vi "Main.vi"() -> ()   [LabVIEW 2018]
uses:
  <vilib>/Instr/_visa.llb/VISA Configure Serial Port (Instr).vi
panel:
  out "Read Count":i32
  out "UART Monitor":string
  out "UART Communication ON/OFF":bool
  in  "VISA resource name":refnum<visa-resource-name>
  in  "Finish Test":bool
  out "Boolean":bool
  in  "Model FLASH Memory":bool
  out "Workspace":string[](array[string])
  out "Tests added to Workspace":i32
  in  "Input":string
  in  "Menu":T1(ring)
  in  "stop":bool
  in  "OK Button":bool
  out "Instructions":string
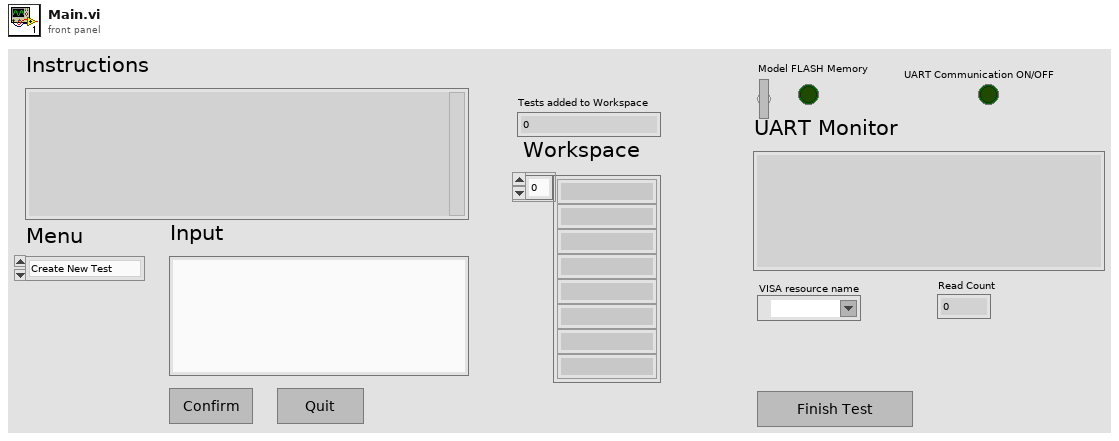
[diagram p1: front panel]
types:
  T1 = enum16{"Create New Test", "Run Single Test", "Run All Tests", "Save Workspace", "Load Workspace", "Delete Test"}
  T2 = enum16{"Inicio", "Create Test A", "Create Test B", "Create Test C", "Create Test D", "Delete Test A", "Delete Test B", "Save", "Load", "Single Test Run", "All Tests Run", "Load Program", "Running Test", "Running Idle", "UART Monitor"}
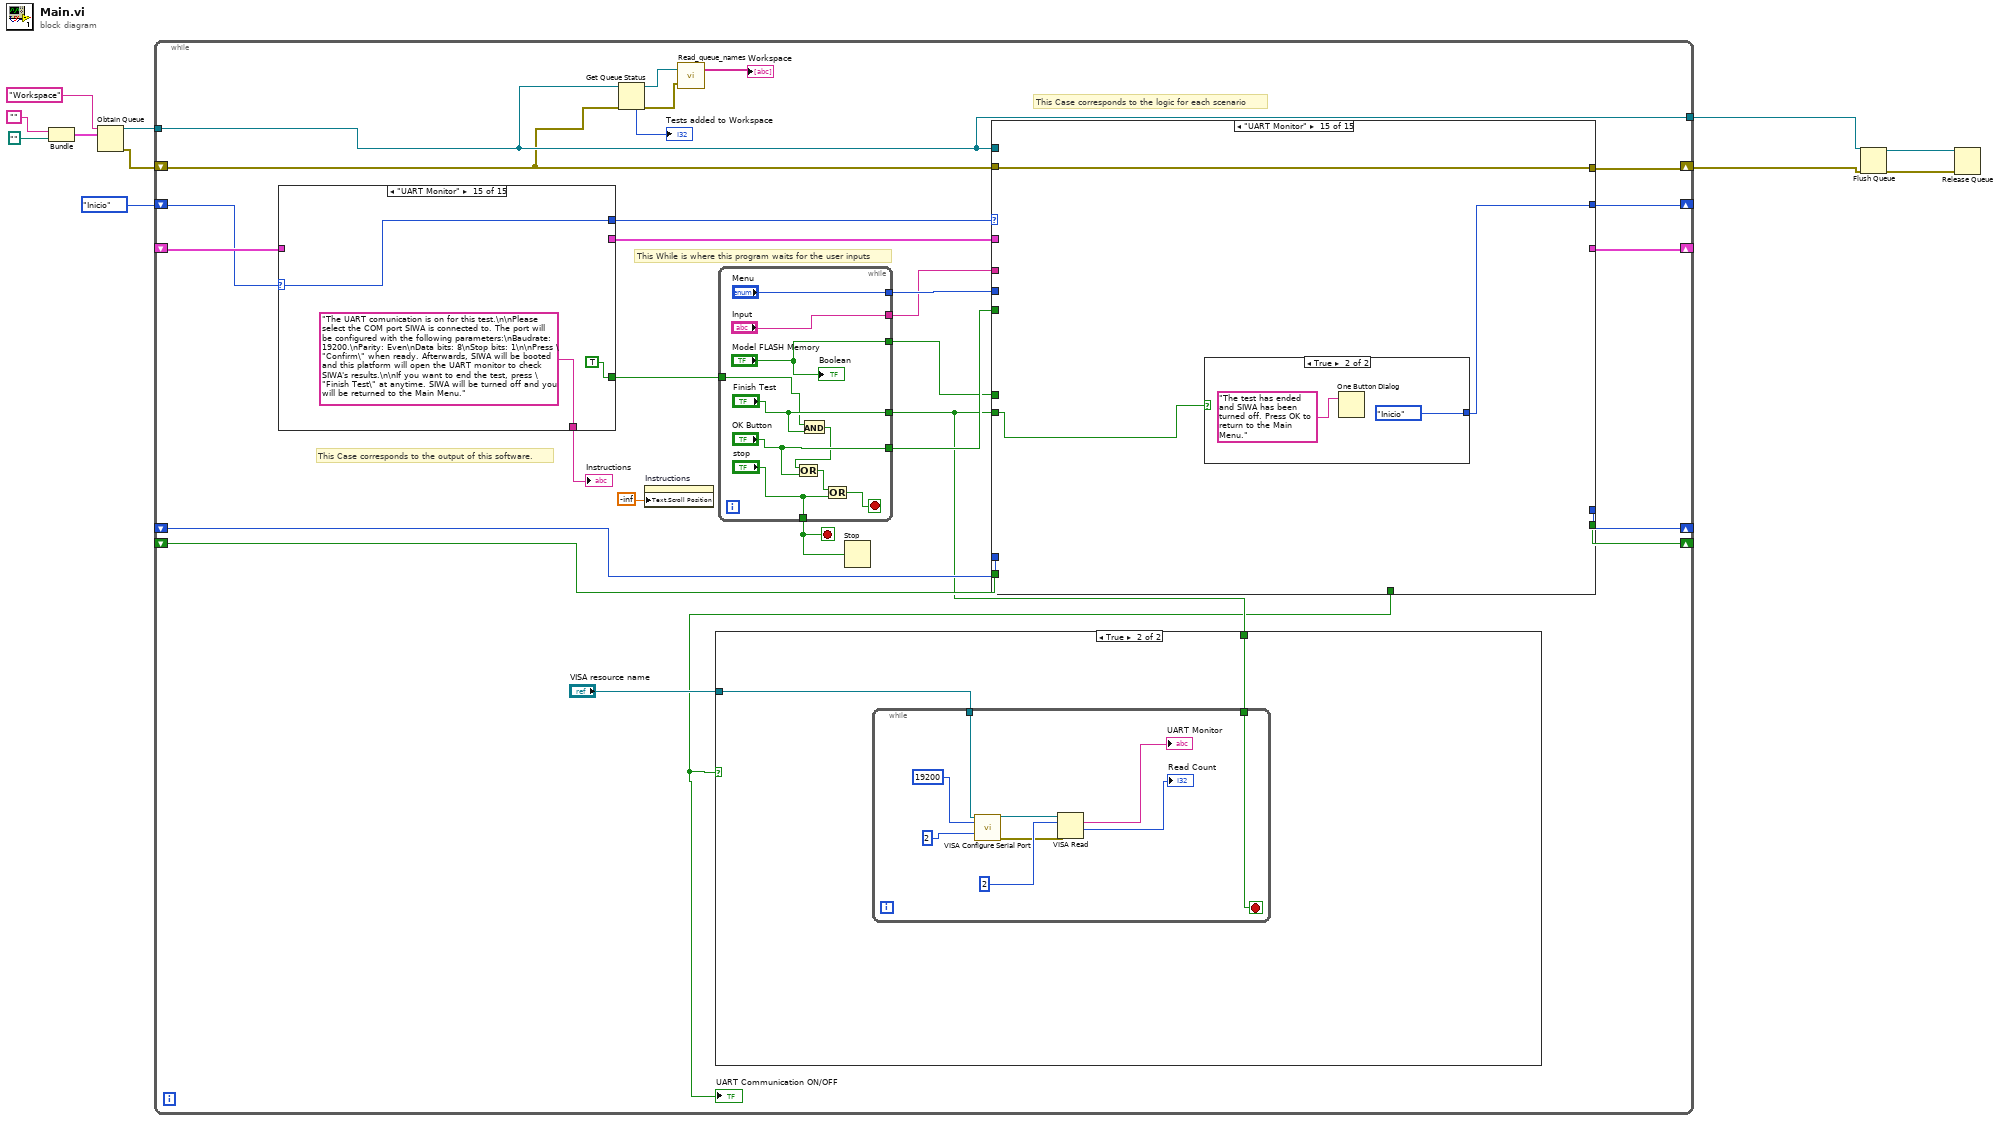
[diagram p0: block diagram]
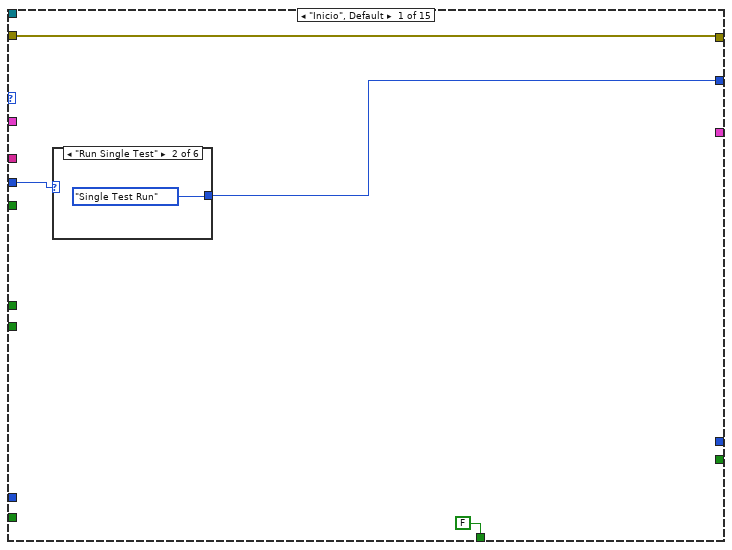
[diagram p3: hidden frame]
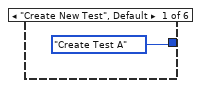
[diagram p4: hidden frame]
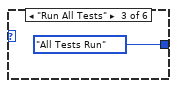
[diagram p5: hidden frame]
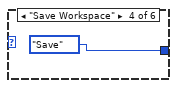
[diagram p6: hidden frame]
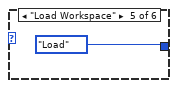
[diagram p7: hidden frame]
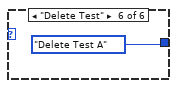
[diagram p8: hidden frame]
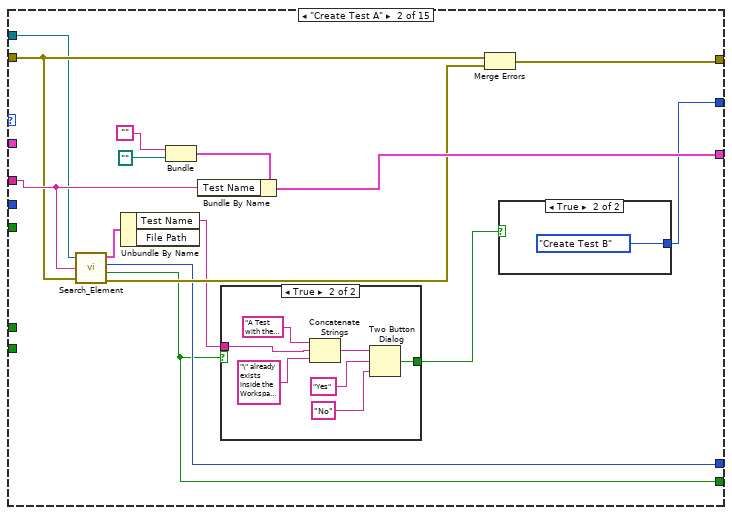
[diagram p9: hidden frame]
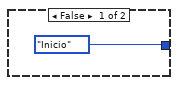
[diagram p10: hidden frame]
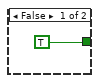
[diagram p11: hidden frame]
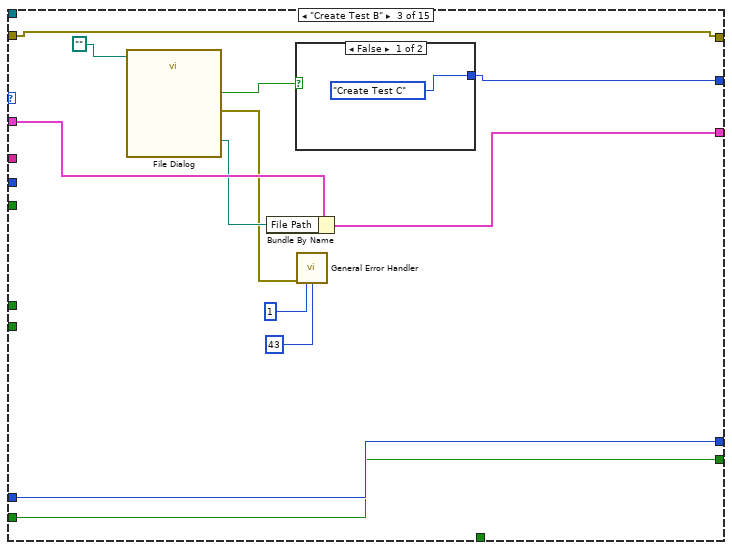
[diagram p12: hidden frame]
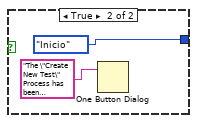
[diagram p13: hidden frame]
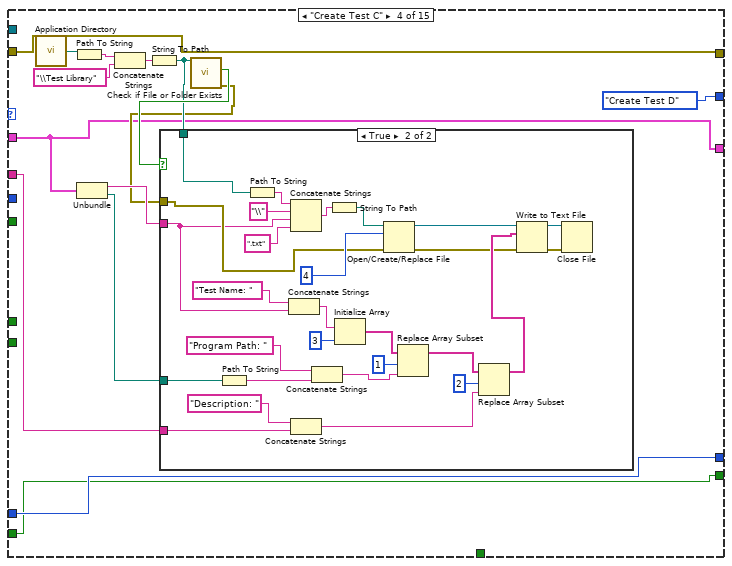
[diagram p14: hidden frame]
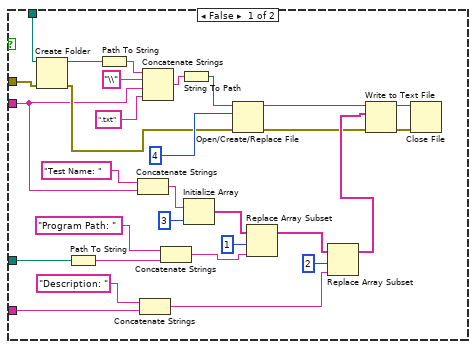
[diagram p15: hidden frame]
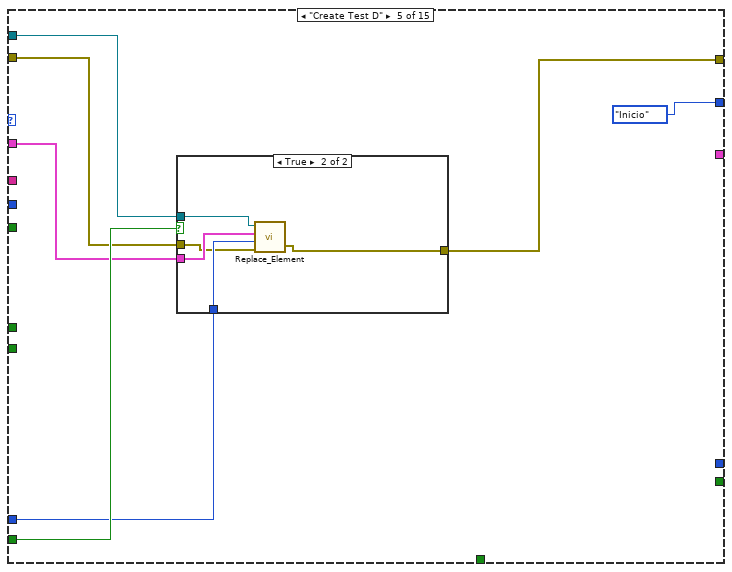
[diagram p16: hidden frame]
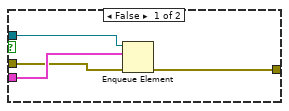
[diagram p17: hidden frame]
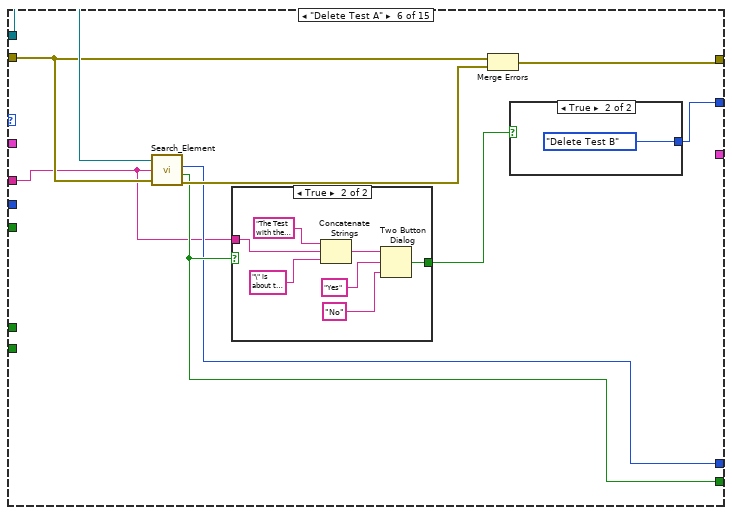
[diagram p18: hidden frame]
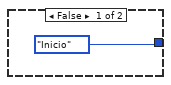
[diagram p19: hidden frame]
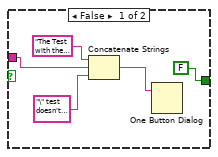
[diagram p20: hidden frame]
diagram:
  n1 = Bundle("Test Name"="", "File Path"=path "") -> (w9:cluster{"Test Name":string, "File Path":path})  [unwired: 1 in]
  n2 = Obtain Queue(name (unnamed)="Workspace", element data type=w9) -> (queue out=w3:refnum<queue>, error out=w7:errorcluster)  [unwired: 3 in, 1 out]
  n3 = while {
    shift-right: [w32] -> _
    shift-left: _ -> [w33]
    shift-right: [w31] -> w6
    shift-left: w7 -> [w25]
    tunnel: w3 -> [w26]
    tunnel: [w26] -> w2
    shift-right: [w24] -> _
    shift-left: _ -> [w23]
    shift-right: [w22] -> _
    shift-left: _ -> [w21]
    shift-right: [w16] -> _
    shift-left: T2."Inicio" -> [w17]
    stop <- w19 stop-if-true
    # "This While is where this program waits for the user inputs"
    # "This Case corresponds to the logic for each scenario"
    # "This Case corresponds to the output of this software."
    n4 = case shown="\"UART Monitor\"" w17 {
      selector: w17 -> [w284 w287 w289 w292 w296 w297 w300 w301 w303 w305 w307 w309 w313 w319 w322]
      tunnel: ["Welcome. This is the Test Environment designed for SIWA.\nSelect which kind of operation do you want to run from the Menu." "Please write below a name for this new test. If the Test File already exists inside the Test Library, it will be overwritted.\n\nThen, press \"Confirm\" to continue." "Now, attach a Program File to this new test. The selected Program File will be the main program loaded in SIWA each time you run this test in the future.\n\nPress \"Confirm\" to continue and select the desired Program File. Press \"OK\" afterwards.\n\nIMPORTANT: The Program File is a .txt file, where each line is a Disassembled 32-bit RISCV Instruction (RV32I format) written in Hexadecimal Code. Please be sure that the selected Program File is constructed in a similar fashion. Otherwise, the test could run into errors." "Write a brief description for this new test.\n\nThe description introduced below will be added to the Test File. That way, it will be easier to understand whatever this test does.\n\nPress Confirm when the description is finished." "The Test File has been created and added to the Testbench succesfully.\n\nYou can find the Test File inside the Test Library folder as <Testname>.txt.\n\nPress Confirm the return to the Main Menu.\n\n" "Introduce the name of the Test you want to remove from the Workspace.\n\nNote: This process won't delete the Test File from your computer. If you wish to delete it completely, it is recommended to do it manually. All tests are stored inside the Test Library file.\n\nPress \"Confirm\" to return to continue." "The selected Test has been succesfully removed from the Workspace.\n\nPress \"Confirm\" to return to the Main Menu." "This feature is still under development.\nPress \"Confirm\" to return to the Main Menu." "This feature is still under development.\nPress \"Confirm\" to return to the Main Menu." "Write the name of the Test you wish to run on SIWA.\n\nPress \"Confirm\" to continue." "This feature is still under development.\nPress \"Confirm\" to return to the Main Menu." "The selected programmed has been loaded inside the FPGA and is ready to be booted on SIWA.\n\nPress \"Confirm\" to boot SIWA.\n\nPress \"Finish Test\" to cancel and return to the Main Menu." "The UART comunication is off for this test. From now on, this platform is indefinitly on an idle state while SIWA is running the loaded program.\n\nIf you want to end the test, press \"Finish Test\". SIWA will be turned off and you will be returned to the Main Menu." w316 "The UART comunication is on for this test.\n\nPlease select the COM port SIWA is connected to. The port will be configured with the following parameters:\nBaudrate: 19200.\nParity: Even\nData bits: 8\nStop bits: 1\n\nPress \"Confirm\" when ready. Afterwards, SIWA will be booted and this platform will open the UART monitor to check SIWA's results.\n\nIf you want to end the test, press \"Finish Test\" at anytime. SIWA will be turned off and you will be returned to the Main Menu."] -> w39
      tunnel: [w284 w287 w289 w292 w296 w297 w300 w301 w303 w305 w307 w309 w313 w319 w322] -> w38
      tunnel: [_ _ w288 w291 w294 _ _ _ _ _ _ _ _ w314 _] -> w34
      tunnel: w33 -> [_ _ w288 w291 w294 _ _ _ _ _ _ _ _ w314 _]
      tunnel: [FALSE _ _ _ _ _ _ _ _ _ _ _ TRUE _ TRUE] -> w12
      frame "Inicio", Default {
      }
      frame "Create Test A" {
      }
      frame "Create Test B" {
      }
      frame "Create Test C" {
      }
      frame "Create Test D" {
      }
      frame "Delete Test A" {
      }
      frame "Delete Test B" {
      }
      frame "Save" {
      }
      frame "Load" {
      }
      frame "Single Test Run" {
      }
      frame "All Tests Run" {
      }
      frame "Running Test" {
      }
      frame "Running Idle" {
      }
      frame "Load Program" {
        n5 = Unbundle By Name(w314) -> ("Test Name"=w315:string)  [unwired: 1 out]
        n6 = Concatenate Strings("The Test with the name \"", w315, "\" test has been selected. The Program File attached to it will be loaded into SIWA.\n\nPress \"Confirm\" to continue.") -> (w316:string)
      }
      frame "UART Monitor" {
      }
    }
    "Instructions" <- w39
    n7 = Get Queue Status(queue=w26, error in (no error)=w25) -> (queue out=w28:refnum<queue>, error out=w20:errorcluster, # elements in queue=→"Tests added to Workspace":i32)  [unwired: 1 in, 5 out]
    n8 = property on="Instructions" class="Str"("Text.Scroll Position"=-inf) -> ()  [unwired: 2 in, 2 out]
    n9 = call "Read_queue_names.vi"("error in (no error)"=w20, "Queue in"=w28) -> ("Array"=→"Workspace":string[])  [unwired: 1 out]
    n10 = while {
      tunnel: ["OK Button"] -> w37
      tunnel: ["stop"] -> w19
      tunnel: ["Menu"] -> w36
      tunnel: ["Input"] -> w35
      tunnel: ["Model FLASH Memory"] -> w18
      tunnel: ["Finish Test"] -> w14
      tunnel: w12 -> [w274]
      stop <- w282 stop-if-true
      n11 = And(x=w274, y="Finish Test") -> (x .and. y?=w273:bool)
      n12 = Or(x=w273, y="OK Button") -> (x .or. y?=w276:bool)
      n13 = Or(x=w276, y="stop") -> (x .or. y?=w282:bool)
      "Boolean" <- "Model FLASH Memory"
    }
    n14 = Stop(stop? (T)=w19) -> ()
    n15 = case shown="\"UART Monitor\"" w38 {
      tunnel: w37 -> [_ _ _ _ _ _ _ _ _ _ _ _ _ _ _]
      tunnel: w36 -> [w54 _ _ _ _ _ _ _ _ _ _ _ _ _ _]
      tunnel: w35 -> [_ w71 _ w108 _ w191 _ _ _ w223 _ _ _ _ _]
      tunnel: w34 -> [_ _ w96 w105 w178 _ _ _ _ _ _ _ _ w265 _]
      tunnel: [_ w72 w94 w105 _ _ _ _ _ w224 _ _ _ _ _] -> w32
      tunnel: [w53 w68 w93 w104 w177 w194 w215 w219 w221 w227 w239 w245 w250 w266 w269] -> w31
      tunnel: w25 -> [w53 w70 w93 w104 w176 w195 w216 w219 w221 w228 w239 w245 w250 w266 w269]
      tunnel: w26 -> [_ w64 _ _ w179 w196 w217 _ _ w229 _ _ _ _ _]
      tunnel: [_ w66 w88 w103 _ w192 _ _ _ _ _ _ _ _ _] -> w24
      tunnel: w23 -> [_ _ w88 w103 w175 _ w214 _ _ _ _ _ _ _ _]
      tunnel: [_ w65 w87 w102 _ w193 _ _ _ _ _ _ _ _ _] -> w22
      tunnel: w21 -> [_ _ w87 w102 w180 _ _ _ _ _ _ _ _ _ _]
      tunnel: w18 -> [_ _ _ _ _ _ _ _ _ _ _ _ _ w255 _]
      tunnel: [w52 w61 w86 T2."Create Test D" T2."Inicio" w190 T2."Inicio" T2."Inicio" T2."Inicio" w222 T2."Inicio" w241 w248 T2."Running Test" w267] -> w16
      tunnel: w14 -> [_ _ _ _ _ _ _ _ _ _ _ _ w249 _ w268]
      tunnel: [FALSE _ _ _ _ _ _ _ _ _ _ w240 _ _ _] -> w13
      frame "Inicio", Default {
        n16 = case shown="\"Run Single Test\"" w54 {
          tunnel: [T2."Create Test A" T2."Single Test Run" T2."All Tests Run" T2."Save" T2."Load" T2."Delete Test A"] -> w52
          frame "Create New Test", Default {
          }
          frame "Run Single Test" {
          }
          frame "Run All Tests" {
          }
          frame "Save Workspace" {
          }
          frame "Load Workspace" {
          }
          frame "Delete Test" {
          }
        }
      }
      frame "Create Test A" {
        n17 = call "Search_Element.vi"("Queue in"=w64, "String"=w71, "error in (no error)"=w70) -> ("cluster"=w63:cluster{"Test Name":string, "File Path":path}, "Numeric"=w66:i32, "Boolean"=w65:bool, "error out"=w69:errorcluster)
        n18 = Unbundle By Name(w63) -> ("Test Name"=w62:string)  [unwired: 1 out]
        n19 = Bundle("Test Name"="", "File Path"=path "") -> (w73:cluster{"Test Name":string, "File Path":path})  [unwired: 1 in]
        n20 = Bundle By Name(cluster=w73, "Test Name"=w71) -> (w72:cluster{"Test Name":string, "File Path":path})
        n21 = case shown="True" w65 {
          tunnel: w62 -> [_ w83]
          tunnel: [TRUE w79] -> w67
          frame False {
          }
          frame True {
            n22 = Concatenate Strings("A Test with the name \"", w83, "\" already exists inside the Workspace.\n\nDo you wish to overwrite the existing Test with the new one?\n\n(If No, then you will be redirected to the Main Menu)") -> (w85:string)
            n23 = Two Button Dialog(message=w85, 1:"No", 2:"Yes") -> (T button?=w79:bool)
          }
        }
        n24 = Merge Errors(w70, w69) -> (w68:errorcluster)
        n25 = case shown="True" w67 {
          tunnel: [T2."Inicio" T2."Create Test B"] -> w61
          frame False {
          }
          frame True {
          }
        }
      }
      frame "Create Test B" {
        n26 = call "File Dialog"("start path"=path "") -> ("selected path"=w95:path, "cancelled"=w92:bool, "error out"=w91:errorcluster)  [unwired: 11 in, 1 out]
        n27 = Bundle By Name(cluster=w96, "File Path"=w95) -> (w94:cluster{"Test Name":string, "File Path":path})
        n28 = case shown="False" w92 {
          tunnel: [T2."Create Test C" T2."Inicio"] -> w86
          frame False {
          }
          frame True {
            n29 = One Button Dialog(message="The \"Create New Test\" Process has been canceled. Each test needs a Program File attached to it.") -> ()  [unwired: 1 in, 1 out]
          }
        }
        n30 = call <vilib>:"General Error Handler.vi"("error in (no error)"=w91, "[exception action] (none:0)"=1, "[exception code]"=43) -> ()  [unwired: 8 in, 5 out]
      }
      frame "Create Test C" {
        n31 = call <vilib>:"Application Directory.vi"() -> ("Application Directory"=w106:path)
        n32 = Path To String(path=w106) -> (string=w115:string)
        n33 = Unbundle(w105) -> ("Test Name"=w110:string, "File Path"=w109:path)
        n34 = Concatenate Strings(w115, "\\Test Library") -> (w113:string)
        n35 = String To Path(string=w113) -> (path=w111:path)
        n36 = call <vilib>:"Check if File or Folder Exists.vi"("path"=w111) -> ("error out"=w107:errorcluster, "file or folder exists?"=w112:bool)  [unwired: 8 in, 1 out]
        n37 = case shown="True" w112 {
          tunnel: w111 -> [w145 w150]
          tunnel: w110 -> [w117 w147]
          tunnel: w109 -> [w131 w161]
          tunnel: w108 -> [w126 w156]
          tunnel: w107 -> [w119 w149]
          frame False {
            n38 = Create Folder(path (use dialog)=w145, error in=w119) -> (created path=w142:path, error out=w120:errorcluster)  [unwired: 1 in, 1 out]
            n39 = Path To String(path=w131) -> (string=w130:string)
            n40 = Path To String(path=w142) -> (string=w144:string)
            n41 = Concatenate Strings("Test Name: ", w117) -> (w136:string)
            n42 = Concatenate Strings("Description: ", w126) -> (w125:string)
            n43 = Concatenate Strings(w144, "\\", w117, ".txt") -> (w143:string)
            n44 = Concatenate Strings("Program Path: ", w130) -> (w132:string)
            n45 = String To Path(string=w143) -> (path=w141:path)
            n46 = Initialize Array(w136, 3) -> (w138:string[])
            n47 = Open/Create/Replace File(file path (use dialog)=w141, error in=w120, operation (0:open)=4) -> (refnum out=w139:refnum<file>, error out=w121:errorcluster)  [unwired: 3 in, 1 out]
            n48 = Replace Array Subset(array=w138, new element=w132, index=1) -> (w128:string[])
            n49 = Replace Array Subset(array=w128, new element=w125, index=2) -> (w124:string[])
            n50 = Write to Text File(file (use dialog)=w139, text=w124, error in=w121) -> (refnum out=w122:refnum<file>, error out=w123:errorcluster)  [unwired: 1 in, 1 out]
            n51 = Close File(refnum=w122, error in=w123) -> ()  [unwired: 2 out]
          }
          frame True {
            n52 = Path To String(path=w161) -> (string=w160:string)
            n53 = Path To String(path=w150) -> (string=w173:string)
            n54 = Concatenate Strings("Test Name: ", w147) -> (w166:string)
            n55 = Concatenate Strings(w173, "\\", w147, ".txt") -> (w172:string)
            n56 = Concatenate Strings("Description: ", w156) -> (w155:string)
            n57 = Concatenate Strings("Program Path: ", w160) -> (w162:string)
            n58 = String To Path(string=w172) -> (path=w171:path)
            n59 = Initialize Array(w166, 3) -> (w168:string[])
            n60 = Open/Create/Replace File(file path (use dialog)=w171, error in=w149, operation (0:open)=4) -> (refnum out=w169:refnum<file>, error out=w151:errorcluster)  [unwired: 3 in, 1 out]
            n61 = Replace Array Subset(array=w168, new element=w162, index=1) -> (w158:string[])
            n62 = Replace Array Subset(array=w158, new element=w155, index=2) -> (w154:string[])
            n63 = Write to Text File(file (use dialog)=w169, text=w154, error in=w151) -> (refnum out=w152:refnum<file>, error out=w153:errorcluster)  [unwired: 1 in, 1 out]
            n64 = Close File(refnum=w152, error in=w153) -> ()  [unwired: 2 out]
          }
        }
      }
      frame "Create Test D" {
        n65 = case shown="True" w180 {
          tunnel: w179 -> [w184 w188]
          tunnel: w178 -> [w183 w187]
          tunnel: [w182 w189] -> w177
          tunnel: w176 -> [w181 w185]
          tunnel: w175 -> [_ w186]
          frame False {
            n66 = Enqueue Element(queue=w184, element=w183, error in (no error)=w181) -> (error out=w182:errorcluster)  [unwired: 1 in, 2 out]
          }
          frame True {
            n67 = call "Replace_Element.vi"("error in (no error)"=w185, "Numeric"=w186, "cluster"=w187, "Queue in"=w188) -> ("error out"=w189:errorcluster)  [unwired: 1 out]
          }
        }
      }
      frame "Delete Test A" {
        n68 = call "Search_Element.vi"("Queue in"=w196, "String"=w191, "error in (no error)"=w195) -> ("Numeric"=w192:i32, "Boolean"=w193:bool, "error out"=w198:errorcluster)  [unwired: 1 out]
        n69 = case shown="True" w193 {
          tunnel: [FALSE w208] -> w197
          tunnel: w191 -> [w205 w207]
          frame False {
            n70 = Concatenate Strings("The Test with the name \"", w205, "\" test doesn't exist inside the Workspace. The Delete Test process has been canceled.\n\nPress \"OK\" to continue.") -> (w202:string)
            n71 = One Button Dialog(message=w202) -> ()  [unwired: 1 in, 1 out]
          }
          frame True {
            n72 = Concatenate Strings("The Test with the name \"", w207, "\" is about to be removed.\n\nDo you wish to remove the Test from the Workspace?\n\n(If No, then you will be redirected to the Main Menu)") -> (w212:string)
            n73 = Two Button Dialog(message=w212, 1:"No", 2:"Yes") -> (T button?=w208:bool)
          }
        }
        n74 = Merge Errors(w195, w198) -> (w194:errorcluster)
        n75 = case shown="True" w197 {
          tunnel: [T2."Inicio" T2."Delete Test B"] -> w190
          frame False {
          }
          frame True {
          }
        }
      }
      frame "Delete Test B" {
        n76 = call "Delete_Element.vi"("error in (no error)"=w216, "Numeric"=w214, "Queue in"=w217) -> ("error out"=w215:errorcluster)  [unwired: 1 out]
      }
      frame "Save" {
      }
      frame "Load" {
      }
      frame "Single Test Run" {
        n77 = call "Search_Element.vi"("Queue in"=w229, "String"=w223, "error in (no error)"=w228) -> ("cluster"=w224:cluster{"Test Name":string, "File Path":path}, "Boolean"=w226:bool, "error out"=w227:errorcluster)  [unwired: 1 out]
        n78 = Unbundle By Name(w224) -> ()  [unwired: 2 out]
        n79 = case shown="True" w226 {
          tunnel: [FALSE TRUE] -> w225
          tunnel: w223 -> [w236 _]
          frame False {
            n80 = Concatenate Strings("The Test with the name \"", w236, "\" doesn't exist inside the Workspace. The Single Test Run process has been canceled.\n\nPress \"OK\" to continue.") -> (w234:string)
            n81 = One Button Dialog(message=w234) -> ()  [unwired: 1 in, 1 out]
          }
          frame True {
          }
        }
        n82 = case shown="True" w225 {
          tunnel: [T2."Inicio" T2."Load Program"] -> w222
          frame False {
          }
          frame True {
          }
        }
      }
      frame "All Tests Run" {
      }
      frame "Running Test" {
        n83 = Two Button Dialog(message="Do you want to turn on the UART Monitor for this particular test?", 1:"No", 2:"Yes") -> (T button?=w240:bool)
        n84 = case shown="False" w240 {
          tunnel: [T2."Running Idle" T2."UART Monitor"] -> w241
          frame False {
          }
          frame True {
          }
        }
      }
      frame "Running Idle" {
        n85 = case shown="True" w249 {
          tunnel: [T2."Running Idle" T2."Inicio"] -> w248
          frame False {
          }
          frame True {
            n86 = One Button Dialog(message="The test has ended and SIWA has been turned off. Press OK to return to the Main Menu.") -> ()  [unwired: 1 in, 1 out]
          }
        }
      }
      frame "Load Program" {
        n87 = Unbundle By Name(w265) -> ("File Path"=w261:path)  [unwired: 1 out]
        n88 = Obtain Queue(name (unnamed)="Program", element data type="") -> (queue out=w262:refnum<queue>, error out=w260:errorcluster)  [unwired: 3 in, 1 out]
        n89 = call "Generate_Program_Queue.vi"("error in (no error)"=w260, "File Path"=w261, "Queue in"=w262) -> ("error out"=w258:errorcluster, "Queue out"=w259:refnum<queue>)
        n90 = call "Load_Program.vi"("error in (no error)"=w258, "FLASH"=w255, "Queue in"=w259) -> ("error out"=w256:errorcluster, "Queue out"=w257:refnum<queue>)
        n91 = Release Queue(queue=w257, error in (no error)=w256) -> ()  [unwired: 1 in, 3 out]
      }
      frame "UART Monitor" {
        n92 = case shown="True" w268 {
          tunnel: [T2."UART Monitor" T2."Inicio"] -> w267
          frame False {
          }
          frame True {
            n93 = One Button Dialog(message="The test has ended and SIWA has been turned off. Press OK to return to the Main Menu.") -> ()  [unwired: 1 in, 1 out]
          }
        }
      }
    }
    "UART Communication ON/OFF" <- w13
    n94 = case shown="True" w13 {
      tunnel: "VISA resource name" -> [_ w41]
      tunnel: w14 -> [_ w40]
      frame False {
      }
      frame True {
        n95 = while {
          tunnel: w41 -> [w43]
          tunnel: w40 -> [w42]
          stop <- w42 stop-if-true
          n96 = call-poly "VISA Configure Serial Port"("VISA resource name"=w43, "baud rate (9600)"=19200, "parity (0:none)"=2) -> ("VISA resource name out"=w50:refnum<visa-resource-name>, "error out"=w48:errorcluster)  [unwired: 11 in]
          n97 = VISA Read(VISA resource name=w50, byte count=2, error in (no error)=w48) -> (read buffer=→"UART Monitor":string, return count=→"Read Count":u32)  [unwired: 2 out]
        }
      }
    }
  }
  n98 = Flush Queue(queue=w2, error in (no error)=w6) -> (queue out=w5:refnum<queue>, error out=w4:errorcluster)  [unwired: 1 out]
  n99 = Release Queue(queue=w5, error in (no error)=w4) -> ()  [unwired: 1 in, 3 out]
